vi "read all I64s.vi"(11 "data table in":T1) -> (1 "values":i64[](array[numeric]), 3 "data table out":T1)   [LabVIEW 2013, in "data bus values.lvlib"]
doc: "Reads an entire set of values from the data table."
uses:
  data bus values.lvlib
  data table.ctl
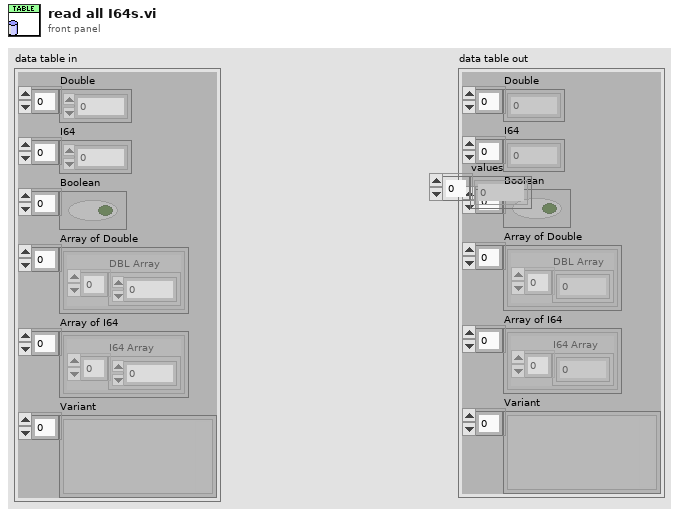
[diagram p1: front panel]
types:
  T1 = typedef "data bus values.lvlib/data table.ctl" = cluster{"Double":dbl[], "I64":i64[], "Boolean":bool[], "Array of Double":cluster{"DBL Array":dbl[]}[], "Array of I64":cluster{"I64 Array":i64[]}[], "Variant":variant[]}
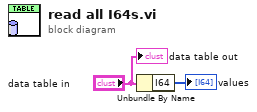
[diagram p0: block diagram]
diagram:
  n1 = Unbundle By Name("data table in") -> ("I64"=→"values":i64[])
  "data table out" <- "data table in"
